vi "复件 随机点新.vi"() -> (0 "输出数组":i32[][](array[numeric]))   [LabVIEW 2014]
panel:
  out "数组":i32[][](array[numeric])
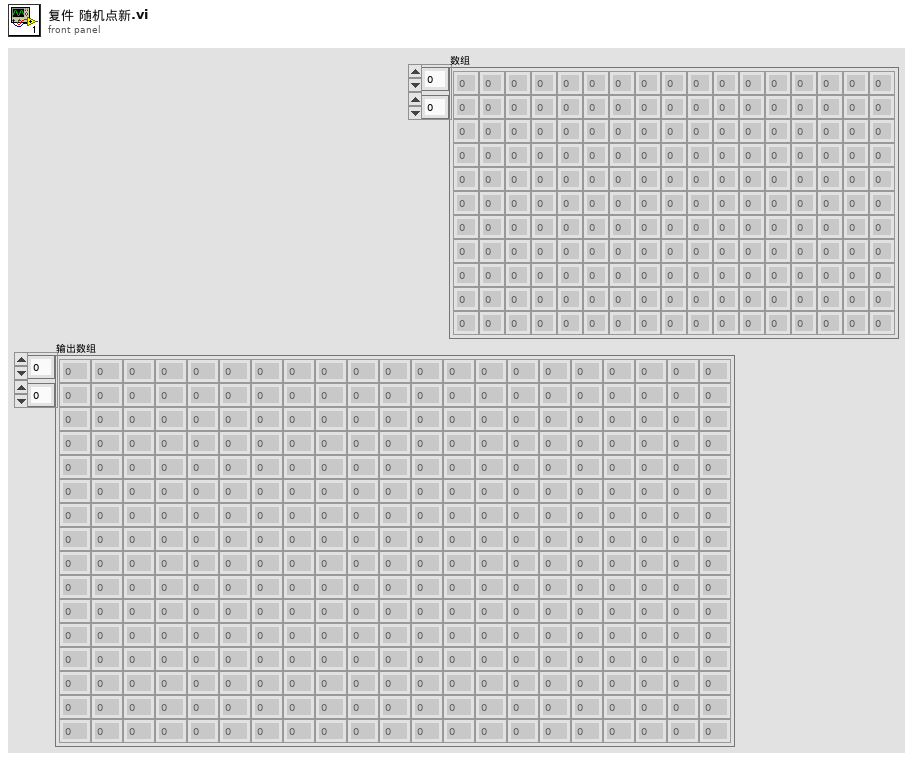
[diagram p1: front panel]
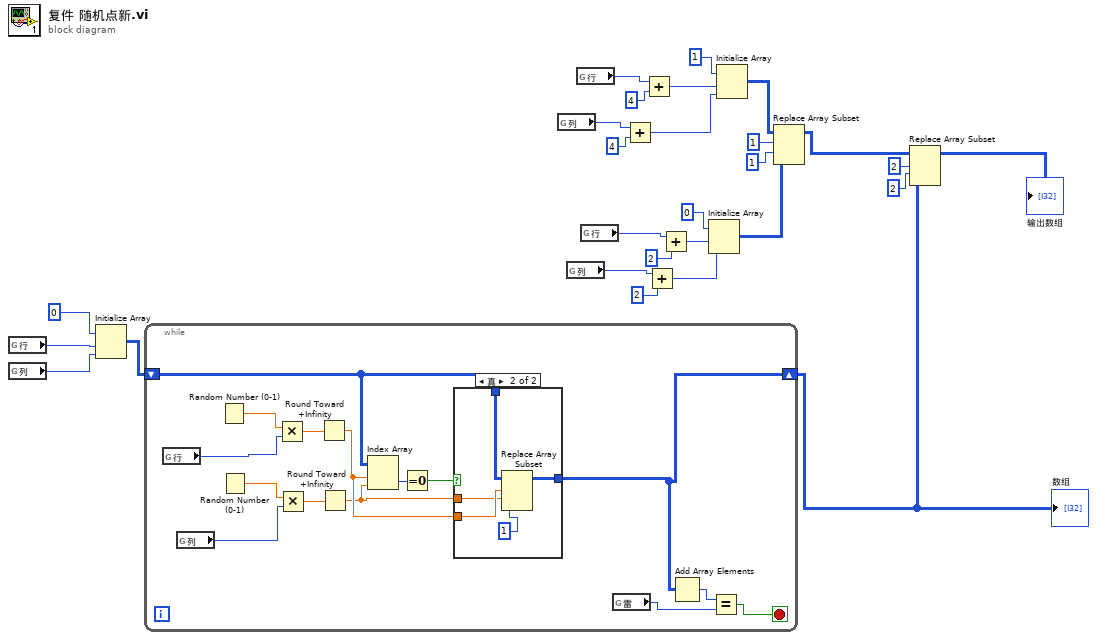
[diagram p0: block diagram]
diagram:
  n1 = global read "全局 1.vi" "行"() -> (w8:i32)
  n2 = global read "全局 1.vi" "列"() -> (w7:i32)
  n3 = Initialize Array(0, w8, w7) -> (w16:i32[][])
  n4 = while {
    shift-right: [w31] -> w15
    shift-left: w16 -> [w36]
    stop <- w32 stop-if-true
    n5 = global read "全局 1.vi" "行"() -> (w28:i32)
    n6 = global read "全局 1.vi" "列"() -> (w29:i32)
    n7 = Random Number (0-1)() -> (number: 0 to 1=w42:dbl)
    n8 = Random Number (0-1)() -> (number: 0 to 1=w40:dbl)
    n9 = Multiply(x=w42, y=w28) -> (x*y=w41:dbl)
    n10 = Multiply(x=w40, y=w29) -> (x*y=w39:dbl)
    n11 = Round Toward +Infinity(x=w41) -> (ceil(x): smallest int >= x=w35:dbl)
    n12 = Round Toward +Infinity(x=w39) -> (ceil(x): smallest int >= x=w34:dbl)
    n13 = Index Array(array=w36, index (row)=w35, index (col)=w34) -> (element=w38:i32)
    n14 = Equal To 0?(x=w38) -> (x = 0?=w37:bool)
    n15 = case shown="真" w37 {
      tunnel: w36 -> [w43 w48]
      tunnel: w35 -> [_ w47]
      tunnel: w34 -> [_ w46]
      tunnel: [w43 w44] -> w31
      frame False {
      }
      frame True {
        n16 = Replace Array Subset(array=w48, new element=1, index (row)=w47, index (col)=w46) -> (w44:i32[][])
      }
    }
    n17 = global read "全局 1.vi" "雷"() -> (w30:i32)
    n18 = Add Array Elements(numeric array=w31) -> (sum=w33:i32)
    n19 = Equal?(x=w33, y=w30) -> (x = y?=w32:bool)
  }
  "数组" <- w15
  n20 = global read "全局 1.vi" "列"() -> (w5:i32)
  n21 = global read "全局 1.vi" "列"() -> (w2:i32)
  n22 = global read "全局 1.vi" "行"() -> (w13:i32)
  n23 = global read "全局 1.vi" "行"() -> (w10:i32)
  n24 = Add(x=w5, y=4) -> (x+y=w4:i32)
  n25 = Add(x=w13, y=4) -> (x+y=w12:i32)
  n26 = Add(x=w2, y=2) -> (x+y=w1:i32)
  n27 = Add(x=w10, y=2) -> (x+y=w9:i32)
  n28 = Initialize Array(0, w9, w1) -> (w22:i32[][])
  n29 = Initialize Array(1, w12, w4) -> (w26:i32[][])
  n30 = Replace Array Subset(array=w26, new element=w22, index (row)=1, index (col)=1) -> (w21:i32[][])
  n31 = Replace Array Subset(array=w21, new element=w15, index (row)=2, index (col)=2) -> (→"输出数组":i32[][])
